vi "Pilot_ON.vi"(7 "State":T2, 8 "error in (no error)":errorcluster, 9 "Data in":T1, 10 "Boiler Controls":refnum<vi>, 11 "Boiler Controls":refnum<vi>) -> (0 "error out":errorcluster, 3 "Data out":T1)   [LabVIEW 2023]
doc: "1_Writes event data log\n2_Turns OFF blinking on Pilot button\n3_Turns ON Natural Gas Valce and Pilot LED\n4_Writes status to Pilot ON"
uses:
  Controls/State.ctl
  Controls/DataCluster.ctl
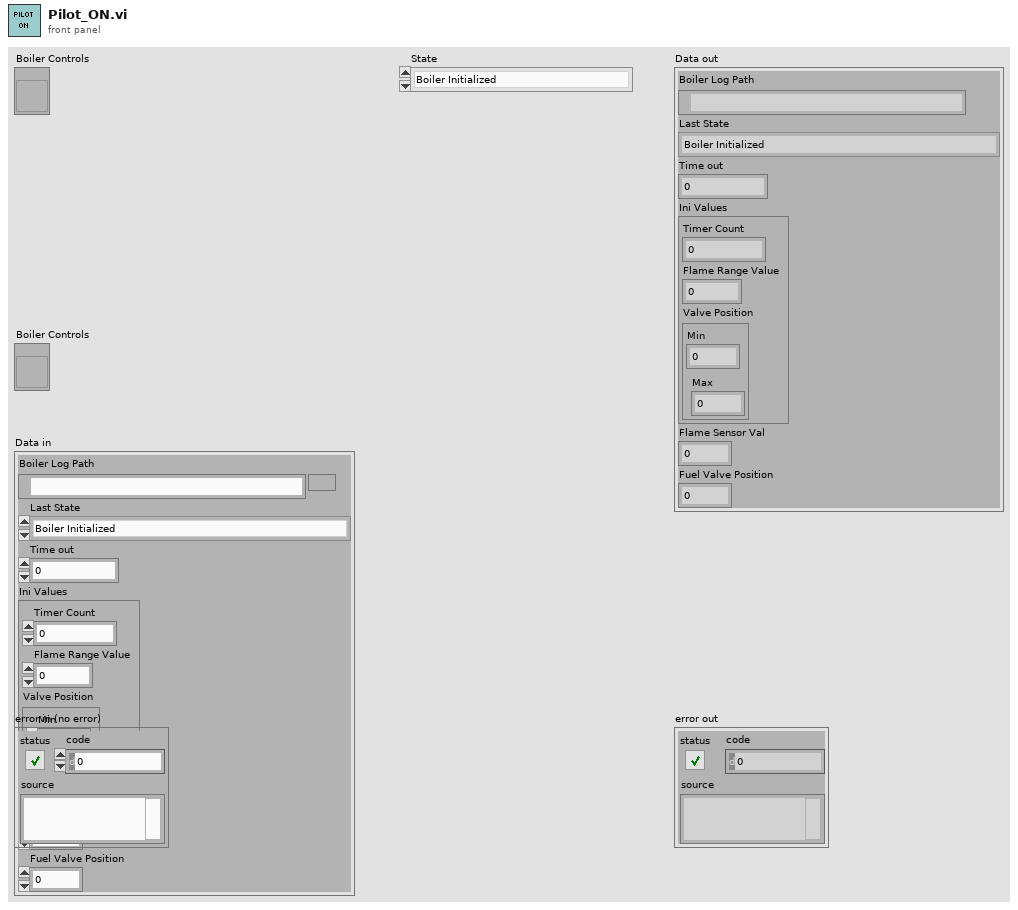
[diagram p1: front panel]
types:
  T1 = typedef "DataCluster.ctl" = cluster{"Boiler Log Path":path, "Last State":T2, "Time out":i32, "Ini Values":cluster{"Timer Count":dbl, "Flame Range Value":dbl, "Valve Position ":cluster{"Min":dbl, "Max":dbl}}, "Flame Sensor Val":dbl, "Fuel Valve Position":dbl}
  T2 = typedef "State.ctl" = enum16{"Boiler Initialized", "Boiler Ready", "Start Pre-Purge", "Pre-Purge Complete", "Pilot On", "Pilot Proved", "Force Draft Fan ON", "Boiler Running", "Start Shutdown Purge", "Shutdown Purge Complete", "Wait for Something"}
  T3 = typedef "Boiler Status Indicators.ctl" = cluster{"Status":string, "Primary Fan":bool, "Natural Gas Valve":bool, "Pilot":bool, "Fuel Valve":bool, "Forced Draft Fan":bool, "Time Count":dbl}
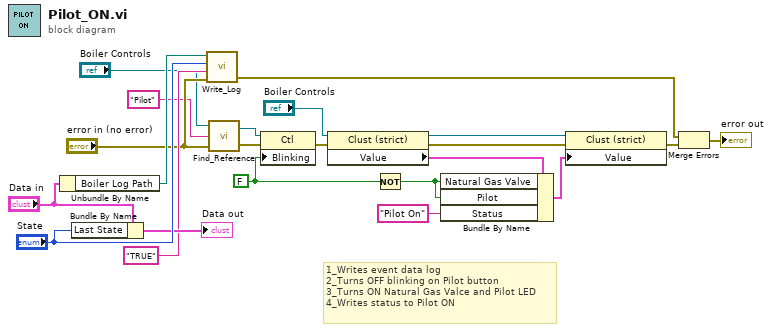
[diagram p0: block diagram]
diagram:
  w16 = FALSE ("Blinking")
  # "1_Writes event data log\n2_Turns OFF blinking on Pilot button\n3_Turns ON Natural Gas Valce and Pilot LED\n4_Writes status to Pilot ON"
  n1 = Unbundle By Name("Data in") -> ("Boiler Log Path"=w15:path)
  n2 = Bundle By Name(cluster="Data in", "Last State"="State") -> (→"Data out":T1)
  n3 = call "Write_Log.vi"("error in (no error)"="error in (no error)", "Event data string"="TRUE", "State"="State", "dup path"=w15) -> ("error out"=w18:errorcluster)  [unwired: 2 in]
  n4 = call "Find_Reference.vi"("error in (no error)"="error in (no error)", "Label"="Pilot", "Cluster in"="Boiler Controls") -> ("error out"=w8:errorcluster, "Ctl Refnum"=w10:refnum<vi>)  [unwired: 1 in]
  n5 = property class="Ctl"(reference=w10, error in=w8, "Blinking"=w16) -> (error out=w9:errorcluster)  [unwired: 1 out]
  n6 = property class="Clust (strict)"(reference="Boiler Controls", error in=w9) -> (reference out=w5:refnum<vi>, error out=w3:errorcluster, "Value"=w6:T3)
  n7 = Not(x=w16) -> (.not. x?=w11:bool)
  n8 = Bundle By Name(cluster=w6, "Natural Gas Valve"=w11, "Pilot"=w11, "Status"="Pilot On") -> (w7:T3)
  n9 = property class="Clust (strict)"(reference=w5, error in=w3, "Value"=w7) -> (error out=w19:errorcluster)  [unwired: 1 out]
  n10 = Merge Errors(w18, w19) -> (→"error out":errorcluster)
